vi "Signal Name Update.vi"(8 "error in (no error)":errorcluster, 11 "Signal Analysis in":refnum<class "Signal Analysis.lvclass">) -> (0 "error out":errorcluster, 3 "Signal Analysis out":refnum<class "Signal Analysis.lvclass">)   [LabVIEW 2023, in "Data Analysis.lvlib" / "Signal Analysis.lvlib" / "Signal Analysis.lvclass"]
uses:
  Signal Analysis.lvclass
  Signal Analysis.lvclass/Signal Analysis.ctl
  Data Analysis.lvlib
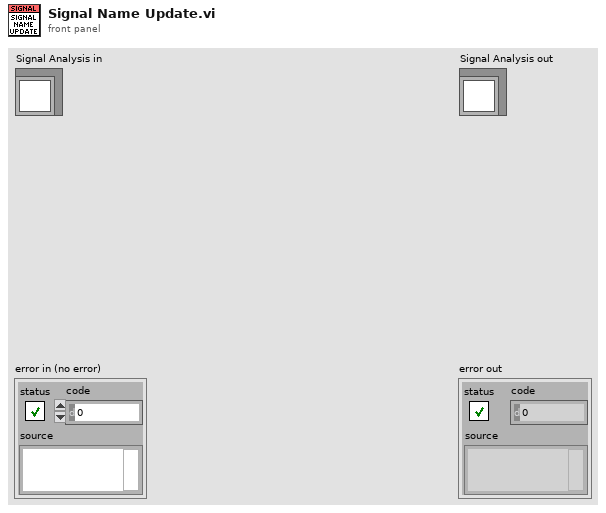
[diagram p1: front panel]
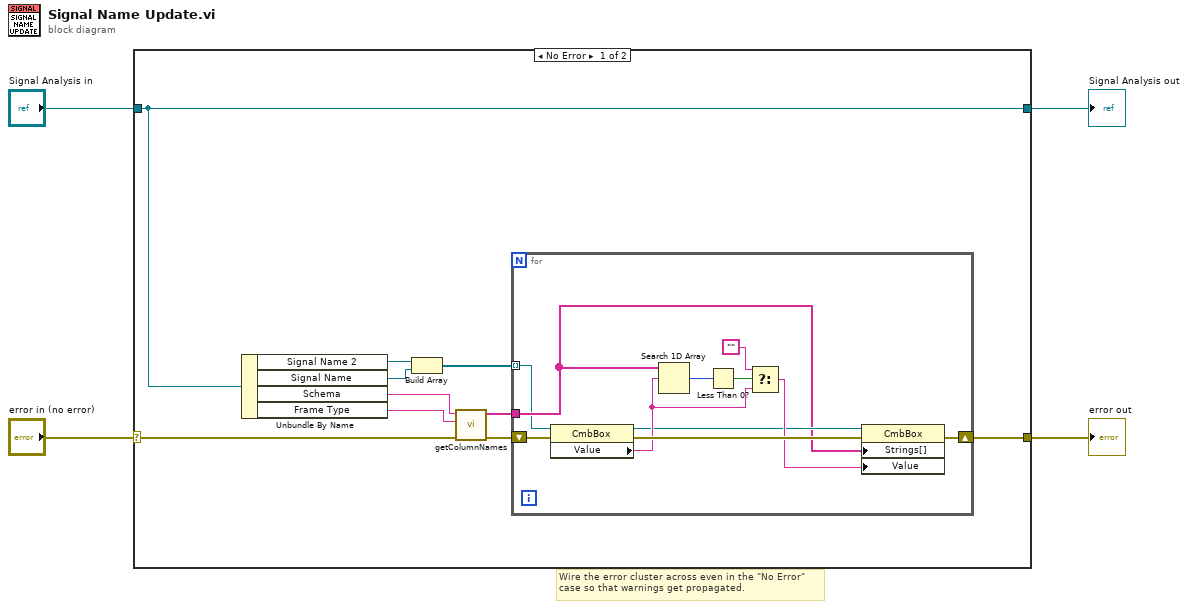
[diagram p0: block diagram]
diagram:
  # "Wire the error cluster across even in the \"No Error\"\ncase so that warnings get propagated."
  n1 = case shown="No Error" "error in (no error)" {
    selector: "error in (no error)" -> [w14 w27]
    tunnel: [w9 w27] -> w3
    tunnel: [w12 w26] -> w1
    tunnel: "Signal Analysis in" -> [w12 w26]
    frame No Error {
      n2 = Unbundle By Name(w12) -> ("Signal Name 2"=w8:refnum<vi>, "Signal Name"=w7:refnum<vi>, "Schema"=w13:string, "Frame Type"=w11:string)
      n3 = Build Array(w8, w7) -> (w5:refnum<vi>[])
      n4 = call "getColumnNames.vi"("error in (no error)"=w14, "tableName"=w11, "schema"=w13) -> ("error out"=w10:errorcluster, "columnNames"=w6:string[])  [unwired: 6 in, 1 out]
      n5 = for {
        shift-right: [w17] -> w9
        shift-left: w10 -> [w18]
        tunnel: w6 -> [w16]
        tunnel: w5 -> [w15] mode=indexing
        n6 = property class="CmbBox"(reference=w15, error in=w18) -> (reference out=w20:refnum<vi>, error out=w25:errorcluster, "Value"=w22:string)
        n7 = Search 1D Array(1D array=w16, element=w22) -> (index of element=w23:i32)  [unwired: 1 in]
        n8 = Less Than 0?(x=w23) -> (x < 0?=w24:bool)
        n9 = Select(t="", s=w24, f=w22) -> (s? t:f=w21:string)
        n10 = property class="CmbBox"(reference=w20, error in=w25, "Strings[]"=w16, "Value"=w21) -> (error out=w17:errorcluster)  [unwired: 1 out]
      }
    }
    frame Error {
    }
  }
  "error out" <- w3
  "Signal Analysis out" <- w1
